vi "Check for Contained Data Type.vi"(6 "LabVIEW class qualified name (\"\")":string, 8 "error in (no error)":errorcluster, 9 "check inside refnums? (F)":bool, 10 "data type to find":T1, 11 "variant":variant) -> (0 "error out":errorcluster, 3 "contains data type to find?":bool)   [LabVIEW 2020, in "NI_Data Type.lvlib"]
doc: "Returns TRUE if <B>variant</B> contains the data type you specify."
uses:
  <vilib>/Utility/Data Type/NI_Data Type.lvlib
  <vilib>/Utility/Data Type/Type Definitions/Data Type.ctl
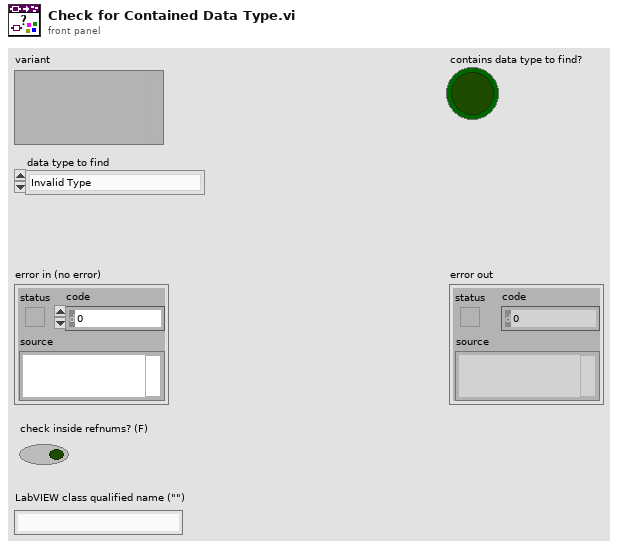
[diagram p1: front panel]
types:
  T1 = typedef "NI_Data Type.lvlib/Data Type.ctl" = enum8{"Invalid Type", "Void", "I8", "I16", "I32", "I64", "U8", "U16", "U32", "U64", "Single Float", "Double Float", "Extended Float", "Single Complex", "Double Complex", "Extended Complex", "Enum U8", "Enum U16", "Enum U32", "Enum U64", "Single Float With Unit", "Double Float With Unit", "Extended Float With Unit", "Single Complex with Unit", "Double Complex with Unit", "Extended Complex with Unit", "Boolean", "String", "Path", "Picture", "Tag", "Array", "Cluster", "Variant", "LV Variant", "Waveform", "Timestamp", "Digital Waveform", "Digital Data", "ExpressData", "Refnum", "External Data", "VI", "Poly VI", "LabVIEW Class Instance", "Fixed Point", "Set Collection", "Map Collection"}
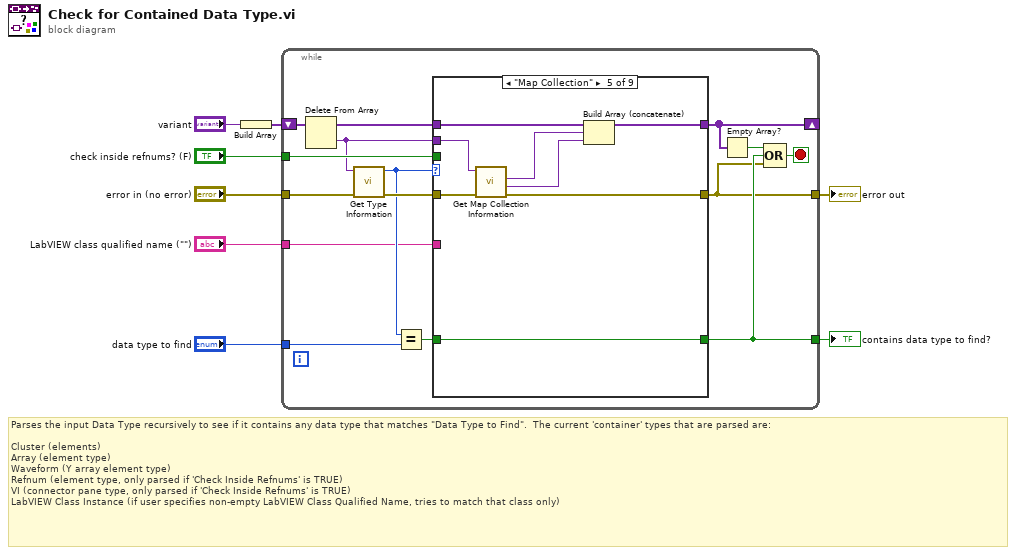
[diagram p0: block diagram]
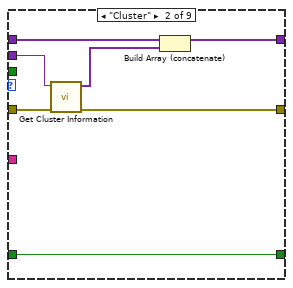
[diagram p3: hidden frame]
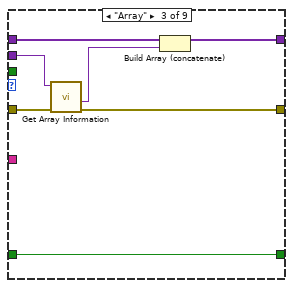
[diagram p4: hidden frame]
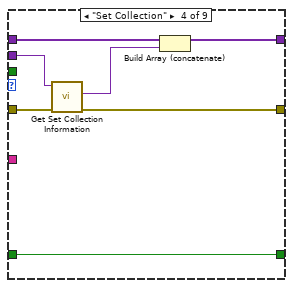
[diagram p5: hidden frame]
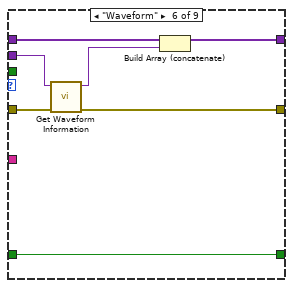
[diagram p6: hidden frame]
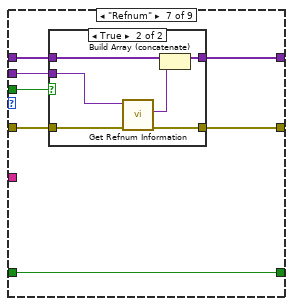
[diagram p7: hidden frame]
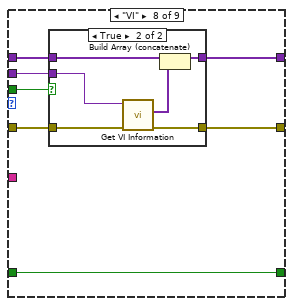
[diagram p9: hidden frame]
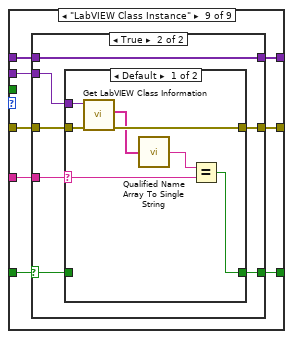
[diagram p11: hidden frame]
diagram:
  # "Parses the input Data Type recursively to see if it contains any data type that matches \"Data Type to Find\".  The current 'container' types that are parsed are:\n\nCluster (elements)\nArray (element type)\nWaveform (Y array element type)\nRefnum (element type, only parsed if 'Check Inside Refnums' is TRUE)\nVI (connector pane type, only parsed if 'Check Inside Refnums' is TRUE)\nLabVIEW Class Instance (if user specifies non-empty LabVIEW Class Qualified Name, tries to match that class only)"
  n1 = Build Array("variant") -> (w2:variant[])
  n2 = while {
    shift-right: [w19] -> _
    shift-left: w2 -> [w23]
    tunnel: [w11] -> w1
    tunnel: "data type to find" -> [w15]
    tunnel: "check inside refnums? (F)" -> [w14]
    tunnel: "LabVIEW class qualified name (\"\")" -> [w13]
    tunnel: "error in (no error)" -> [w22]
    tunnel: [w10] -> w8
    stop <- w17 stop-if-true
    n3 = Delete From Array(array=w23) -> (deleted portion=w9:variant, array with subset deleted=w20:variant[])  [unwired: 2 in]
    n4 = call <vilib>:"Get Type Information.vi"("error in (no error)"=w22, "variant"=w9) -> ("error out"=w21:errorcluster, "type"=w16:T1)  [unwired: 5 in, 3 out]
    n5 = Equal?(x=w16, y=w15) -> (x = y?=w12:bool)
    n6 = case shown="\"Map Collection\"" w16 {
      tunnel: w21 -> [w26 w33 w40 w42 w50 w62 w69 w83 w100]
      tunnel: w20 -> [w25 w31 w37 w47 w55 w59 w67 w81 w94]
      tunnel: [w25 w29 w36 w46 w54 w58 w66 w80 w93] -> w19
      tunnel: [w26 w28 w38 w41 w49 w60 w65 w82 w99] -> w10
      tunnel: w9 -> [_ w32 w39 w44 w52 w61 w68 w79 w97]
      tunnel: w14 -> [_ _ _ _ _ _ w63 w84 _]
      tunnel: w13 -> [_ _ _ _ _ _ _ _ w96]
      tunnel: w12 -> [w24 w27 w34 w45 w53 w56 w64 w78 w95]
      tunnel: [w24 w27 w34 w45 w53 w56 w64 w78 w98] -> w11
      frame Default {
      }
      frame "Cluster" {
        n7 = call <vilib>:"Get Cluster Information.vi"("error in (no error)"=w33, "variant"=w32) -> ("error out"=w28:errorcluster, "cluster elements"=w30:variant[])  [unwired: 8 in]
        n8 = Build Array (concatenate)(w31, w30) -> (w29:variant[])
      }
      frame "Array" {
        n9 = call <vilib>:"Get Array Information.vi"("error in (no error)"=w40, "variant"=w39) -> ("error out"=w38:errorcluster, "array element data type"=w35:variant)  [unwired: 6 in, 2 out]
        n10 = Build Array (concatenate)(w37, w35) -> (w36:variant[])
      }
      frame "Set Collection" {
        n11 = call <vilib>:"Get Set Collection Information.vi"("error in (no error)"=w42, "variant"=w44) -> ("error out"=w41:errorcluster, "element data type"=w43:variant)  [unwired: 8 in]
        n12 = Build Array (concatenate)(w47, w43) -> (w46:variant[])
      }
      frame "Map Collection" {
        n13 = call <vilib>:"Get Map Collection Information.vi"("error in (no error)"=w50, "variant"=w52) -> ("error out"=w49:errorcluster, "value data type"=w48:variant, "key data type"=w51:variant)  [unwired: 7 in]
        n14 = Build Array (concatenate)(w55, w51, w48) -> (w54:variant[])
      }
      frame "Waveform" {
        n15 = call <vilib>:"Get Waveform Information.vi"("error in (no error)"=w62, "variant"=w61) -> ("error out"=w60:errorcluster, "Y array type"=w57:variant)  [unwired: 8 in]
        n16 = Build Array (concatenate)(w59, w57) -> (w58:variant[])
      }
      frame "Refnum" {
        n17 = case shown="True" w63 {
          tunnel: w69 -> [w70 w77]
          tunnel: w68 -> [_ w76]
          tunnel: w67 -> [w71 w75]
          tunnel: [w71 w73] -> w66
          tunnel: [w70 w72] -> w65
          frame False {
          }
          frame True {
            n18 = call <vilib>:"Get Refnum Information.vi"("error in (no error)"=w77, "variant"=w76) -> ("error out"=w72:errorcluster, "strict type"=w74:variant)  [unwired: 6 in, 2 out]
            n19 = Build Array (concatenate)(w75, w74) -> (w73:variant[])
          }
        }
      }
      frame "VI" {
        n20 = case shown="True" w84 {
          tunnel: w83 -> [w86 w92]
          tunnel: [w86 w91] -> w82
          tunnel: w81 -> [w85 w89]
          tunnel: [w85 w88] -> w80
          tunnel: w79 -> [_ w90]
          frame False {
          }
          frame True {
            n21 = call <vilib>:"Get VI Information.vi"("error in (no error)"=w92, "variant"=w90) -> ("error out"=w91:errorcluster, "VI terminal types"=w87:variant[])  [unwired: 6 in, 2 out]
            n22 = Build Array (concatenate)(w89, w87) -> (w88:variant[])
          }
        }
      }
      frame "LabVIEW Class Instance" {
        n23 = case shown="True" w95 {
          selector: w95 -> [w101 w105]
          tunnel: w100 -> [w102 w110]
          tunnel: [w102 w109] -> w99
          tunnel: [w101 w108] -> w98
          tunnel: w97 -> [_ w107]
          tunnel: w96 -> [_ w106]
          tunnel: w94 -> [w103 w104]
          tunnel: [w103 w104] -> w93
          frame False {
          }
          frame True {
            n24 = case shown="Default" w106 {
              selector: w106 -> [w114 _]
              tunnel: w105 -> [_ w118]
              tunnel: [w115 w119] -> w109
              tunnel: w110 -> [w117 w119]
              tunnel: [w113 w118] -> w108
              tunnel: w107 -> [w116 _]
              frame Default {
                n25 = call <vilib>:"Get LabVIEW Class Information.vi"("error in (no error)"=w117, "variant"=w116) -> ("error out"=w115:errorcluster, "qualified LabVIEW class name"=w112:string[])  [unwired: 7 in, 1 out]
                n26 = call <vilib>:"Qualified Name Array To Single String.vi"("Fully Qualified Array"=w112) -> ("Fully Qualified String"=w111:string)
                n27 = Equal?(x=w111, y=w114) -> (x = y?=w113:bool)
              }
              frame "" {
              }
            }
          }
        }
      }
    }
    n28 = Empty Array?(array=w19) -> (empty?=w18:bool)
    n29 = Compound Arithmetic op=OR(w18, w11, w10) -> (w17:bool)
  }
  "contains data type to find?" <- w1
  "error out" <- w8
